vi "Write PID gains.vi"(8 "error in (no error)":errorcluster, 10 "PID gains":T1={"proportional gain (Kc)"=1.0, "integral time (Ti, min)"=0.01, "derivative time (Td, min)"=0.0} {"proportional gain (Kc)" format="%.2f"; "integral time (Ti, min)" format="%.2f"}, 11 "PID Loop in":refnum<class "PID Loop.lvclass">) -> (0 "error out":errorcluster, 3 "PID Loop out":refnum<class "PID Loop.lvclass">)   [LabVIEW 2014, in "PID Loop.lvclass"]
uses:
  PID Loop.lvclass
  PID Gains.ctl
  PID Loop.lvclass/PID Loop.ctl
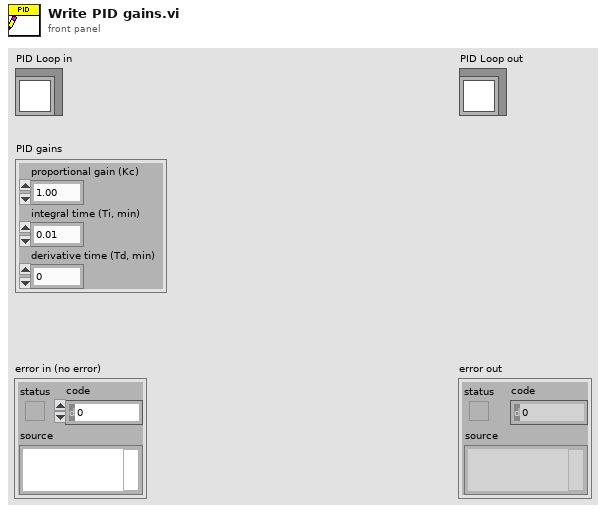
[diagram p1: front panel]
types:
  T1 = typedef "PID Loop.lvclass/PID Gains.ctl" = cluster{"proportional gain (Kc)":dbl, "integral time (Ti, min)":dbl, "derivative time (Td, min)":dbl}
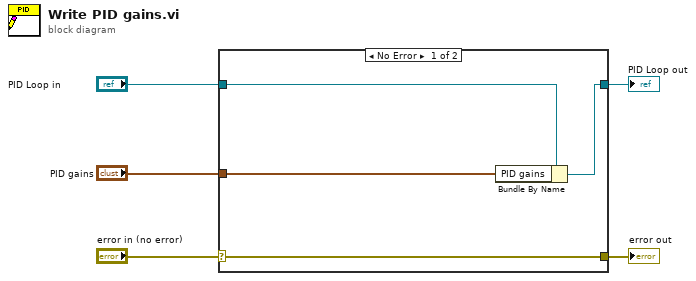
[diagram p0: block diagram]
diagram:
  n1 = case shown="No Error" "error in (no error)" {
    selector: "error in (no error)" -> [w9 w10]
    tunnel: [w9 w10] -> w4
    tunnel: [w7 w11] -> w2
    tunnel: "PID Loop in" -> [w8 w11]
    tunnel: "PID gains" -> [w6 _]
    frame No Error {
      n2 = Bundle By Name(cluster=w8, "PID gains"=w6) -> (w7:refnum<class "PID Loop.lvclass">)
    }
    frame Error {
    }
  }
  "error out" <- w4
  "PID Loop out" <- w2
